vi "Format Tree Rows.vi"(8 "error in":errorcluster, 11 "Tree Ref":refnum<vi>) -> (0 "error out":errorcluster, 3 "Tree Ref out":refnum<vi>)   [LabVIEW 2023]
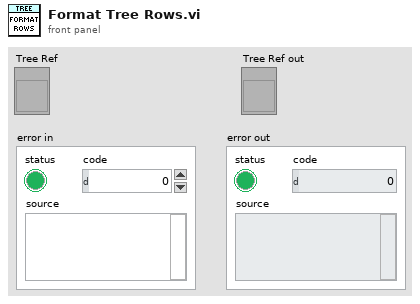
[diagram p1: front panel]
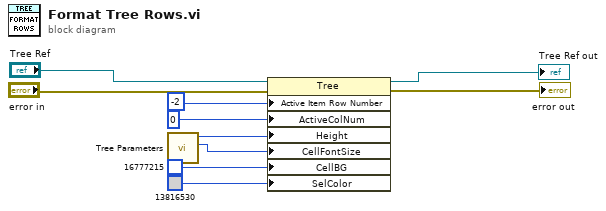
[diagram p0: block diagram]
diagram:
  n1 = call "Tree Parameters.vi"() -> ("Font Size"=w10:i32, "Row Height"=w9:i32)  [unwired: 10 in]
  n2 = property class="Tree"(reference="Tree Ref", error in="error in", "Active Item Row Number"=-2 ("Active Cell:Cell Size:Height"), "ActiveColNum"=0 ("Active Cell:Cell Size:Height"), "Height"=w9, "CellFontSize"=w10, "CellBG"=u32 16777215, "SelColor"=u32 13816530) -> (reference out=→"Tree Ref out":refnum<vi>, error out=→"error out":errorcluster)
